vi "TestExec.Route Check Dialog.vi"(8 "Enable Maint":bool, 10 "This Station's Name":string, 11 "Sta Config File":path) -> ()   [LabVIEW 2018]
uses:
  <vilib>/KATE/Files/File Utils.lvlib
panel:
  out "error IO":errorcluster
  out "Main Tab":enum32{"Operate", "Maint"}(tab)
  out "Active":bool
  out "Status":string
  out "Inbound Process Step":string
  in  "SN":string
  in  "Check Route":bool
  in  "Close":bool
  in  "Go To Maint Tab":bool
  in  "ParamName":string="@SN"
  in  "Go To Route Check tab":bool
  in  "This Station's Route List":string[](array[string])
  in  "Load":bool
  in  "Save As":bool
  in  "Save":bool
  in  "Route Config File":path
  in  "Open Route Config":bool
  in  "Open Station Config":bool
  # "UUT Route Check Utility"
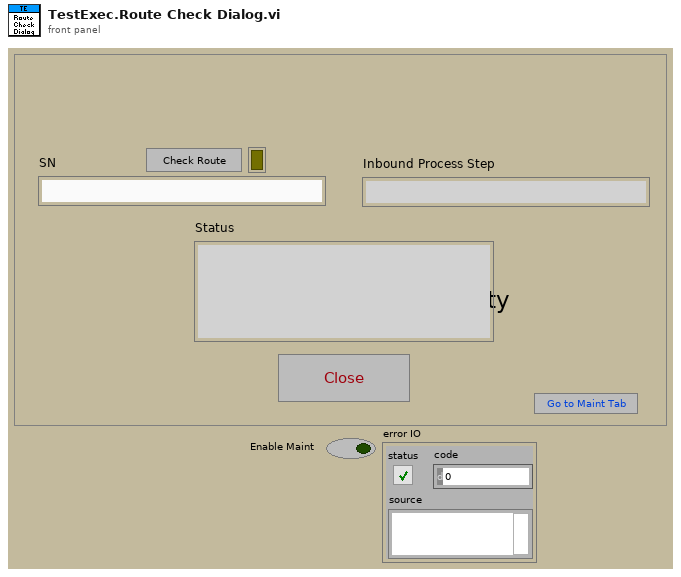
[diagram p1: front panel]
types:
  T1 = enum32{"invalid app kind", "Development System", "Run Time System", "Student Edition", "Embedded LabVIEW", "Evaluation", "Custom"}
  T2 = enum32{"Invalid", "Standard", "Closed", "Hidden", "Minimized", "Maximized"}
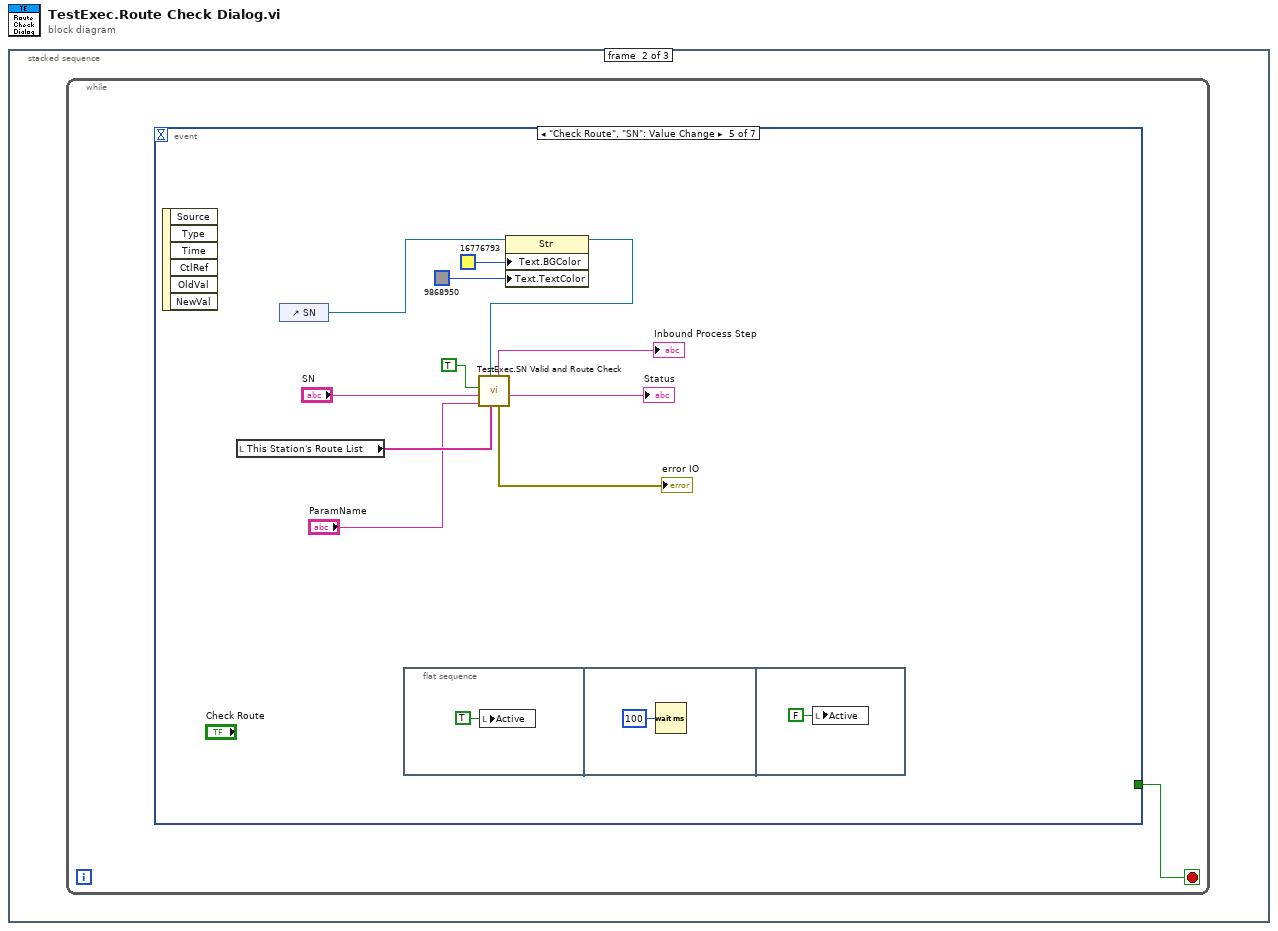
[diagram p0: block diagram]
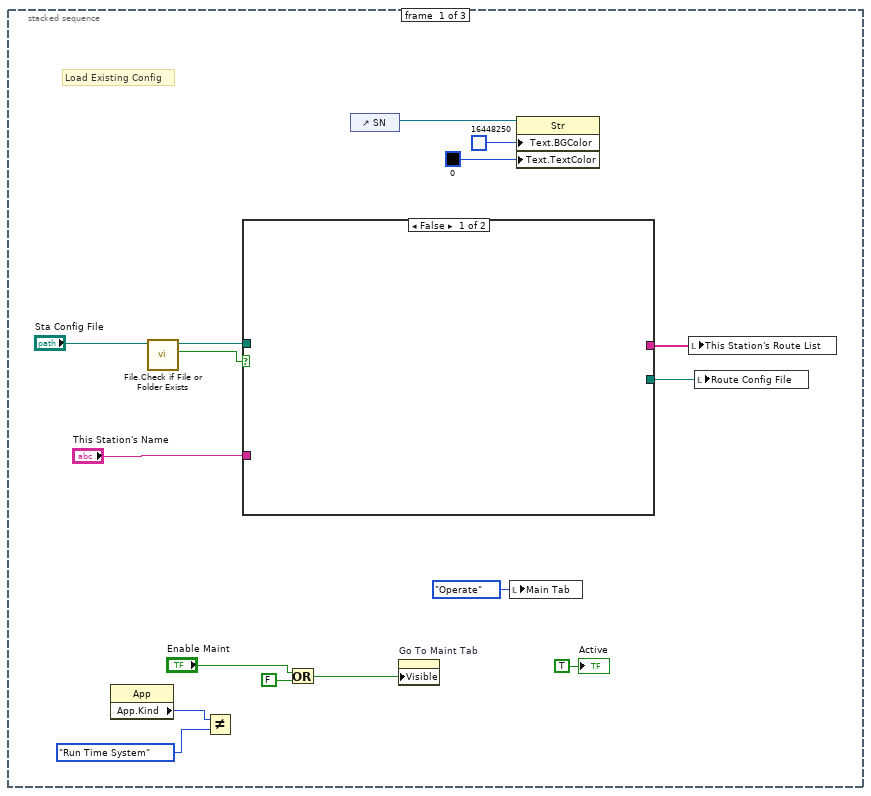
[diagram p2: hidden frame]
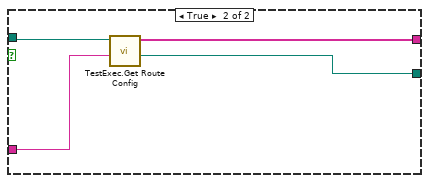
[diagram p3: hidden frame]
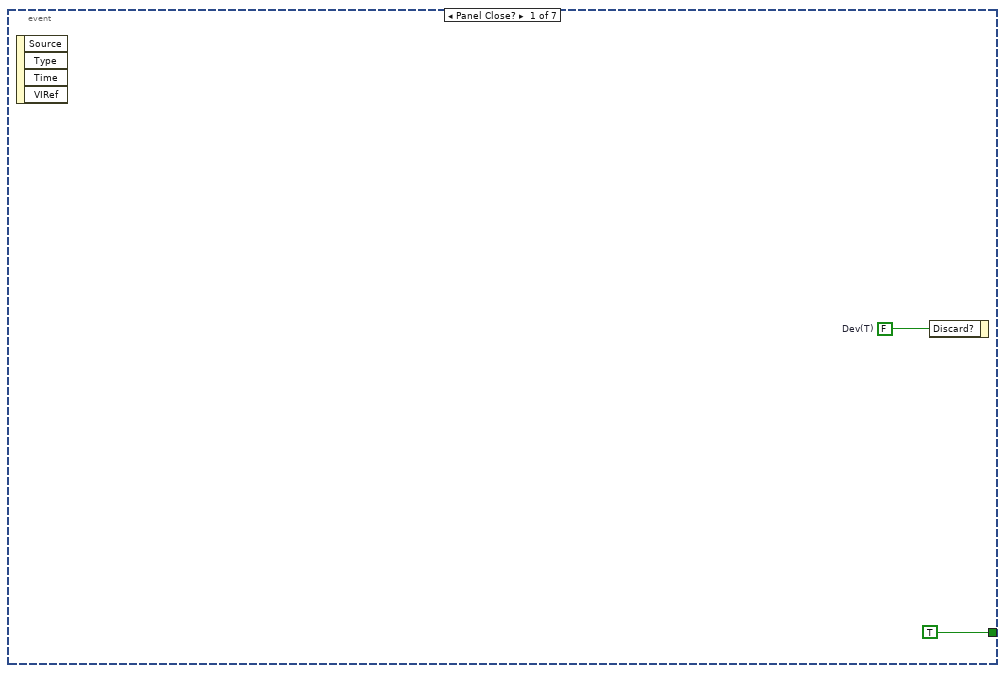
[diagram p4: hidden frame]
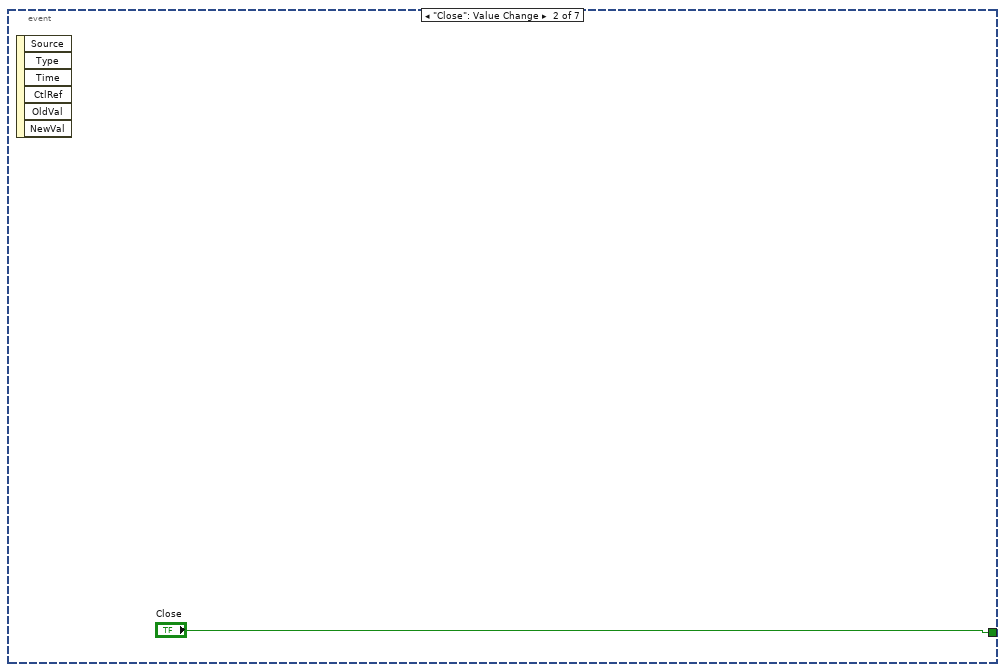
[diagram p5: hidden frame]
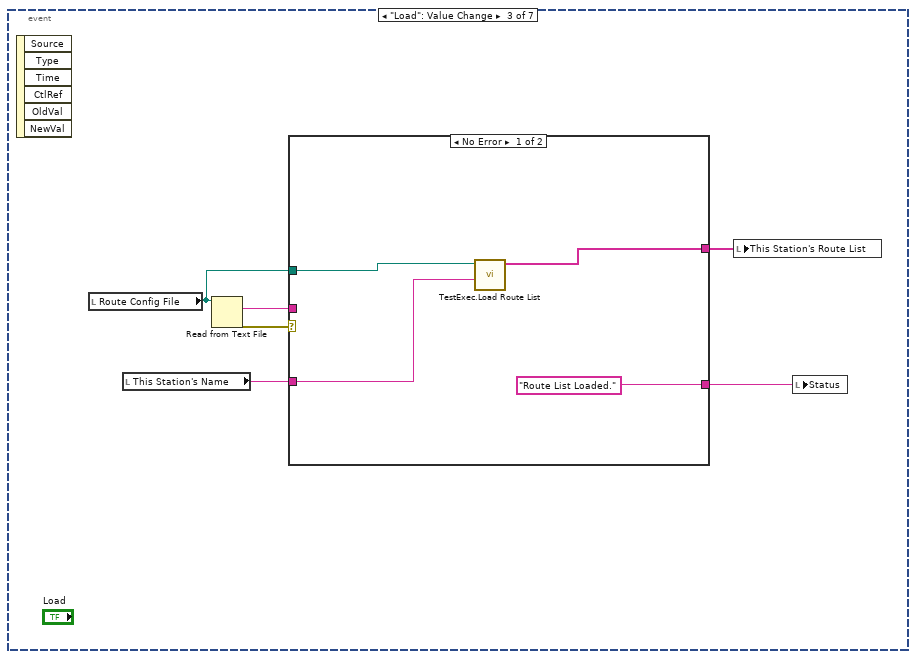
[diagram p6: hidden frame]
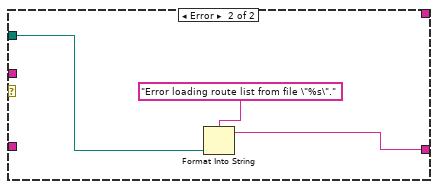
[diagram p7: hidden frame]
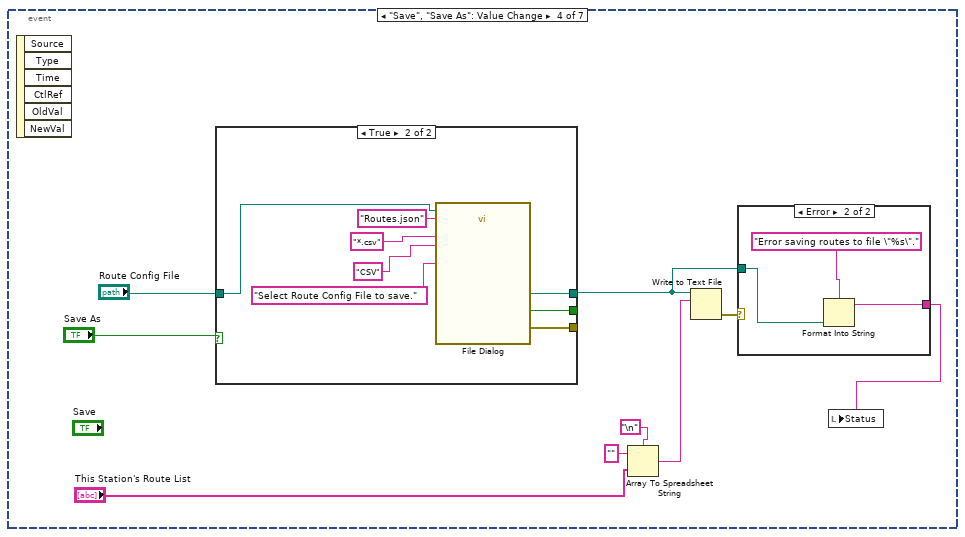
[diagram p8: hidden frame]
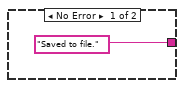
[diagram p9: hidden frame]
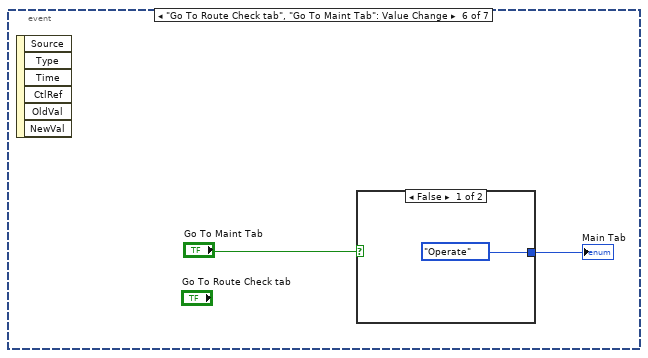
[diagram p11: hidden frame]
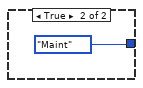
[diagram p12: hidden frame]
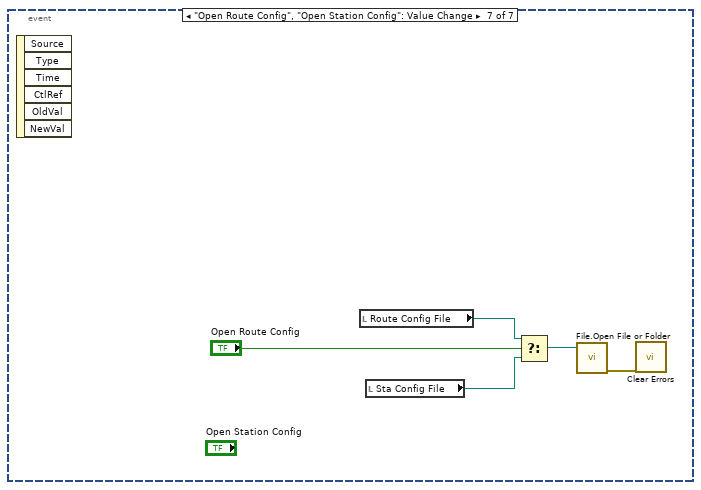
[diagram p13: hidden frame]
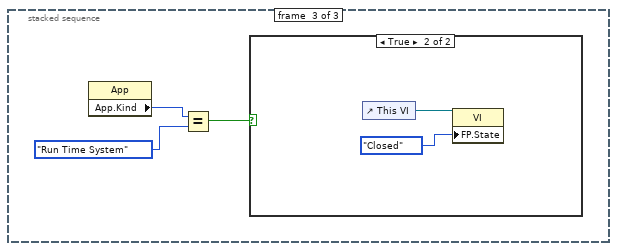
[diagram p14: hidden frame]
diagram:
  n1 = stacked-sequence {
    frame #0 {
      # "Load Existing Config"
      n2 = property class="App"() -> ("App.Kind"=w5:T1)  [unwired: 2 in, 2 out]
      n3 = call <vilib>:"File.Check if File or Folder Exists.vi"("Path"="Sta Config File") -> ("Exists"=w14:bool, "Dup Path"=w15:path)  [unwired: 6 in, 3 out]
      n4 = Not Equal?(x=w5, y=T1."Run Time System" ("Application:Kind")) -> ()  [unwired: 1 out]
      n5 = case shown="False" w14 {
        tunnel: w15 -> [_ w20]
        tunnel: [_ w19] -> w13
        tunnel: [_ w18] -> w12
        tunnel: "This Station's Name" -> [_ w17]
        frame False {
        }
        frame True {
          n6 = call "TestExec.Get Route Config.vi"("Station Name"=w17, "Sta Config INI"=w20) -> ("Route File"=w19:path, "Routes"=w18:string[])  [unwired: 7 in, 1 out]
        }
      }
      n7 = Or(x="Enable Maint", y=FALSE) -> (x .or. y?=w3:bool)
      n8 = control-ref of="SN"() -> (w9:refnum<vi>)
      n9 = property on="Go To Maint Tab" class="Bool"("Visible"=w3) -> ()  [unwired: 2 in, 2 out]
      n10 = local write "Main Tab"(enum32{"Operate", "Maint"}."Operate" ("Main Tab")) -> ()
      n11 = property class="Str"(reference=w9, "Text.BGColor"=u32 16448250, "Text.TextColor"=u32 0) -> ()  [unwired: 1 in, 2 out]
      n12 = local write "This Station's Route List"(w12) -> ()
      n13 = local write "Route Config File"(w13) -> ()
      "Active" <- TRUE ("Active")
    }
    frame #1 {
      n14 = while {
        stop <- w21 stop-if-true
        n15 = event shown="[4] \"Check Route\", \"SN\": Value Change" {
          selector: _ -> [_ _ _ _ _ _ _]
          dyn-events: _ -> [_ _ _ _ _ _ _]
          timeout: _ -> [_ _ _ _ _ _ _]
          tunnel: [TRUE "Close" _ _ _ _ _] -> w21
          event Panel Close? {
            w22 = FALSE  # Dev(T)
            n16 = event-data() -> ()  [unwired: 1 in, 4 out]
            n17 = event-data("Discard?"=w22) -> ()  [unwired: 1 in, 1 out]
          }
          event "Close": Value Change {
            n18 = event-data() -> ()  [unwired: 1 in, 6 out]
          }
          event "Load": Value Change {
            n19 = event-data() -> ()  [unwired: 1 in, 6 out]
            n20 = local read "Route Config File"() -> (w26:path)
            n21 = local read "This Station's Name"() -> (w25:string)
            n22 = Read from Text File(file (use dialog)=w26) -> (text=w30:string, error out=w28:errorcluster)  [unwired: 3 in, 2 out]
            n23 = case shown="No Error" w28 {
              tunnel: w30 -> [_ _]
              tunnel: [w33 _] -> w29
              tunnel: ["Route List Loaded." w36] -> w27
              tunnel: w26 -> [w32 w35]
              tunnel: w25 -> [w31 _]
              frame No Error {
                n24 = call "TestExec.Load Route List.vi"("Station Name"=w31, "Route List File"=w32) -> ("Route List"=w33:string[])  [unwired: 9 in]
              }
              frame Error {
                n25 = Format Into String(format string="Error loading route list from file \"%s\".", w35) -> (resulting string=w36:string)  [unwired: 2 in, 1 out]
              }
            }
            n26 = local write "This Station's Route List"(w29) -> ()
            n27 = local write "Status"(w27) -> ()
          }
          event "Save", "Save As": Value Change {
            n28 = event-data() -> ()  [unwired: 1 in, 6 out]
            n29 = case shown="True" "Save As" {
              tunnel: [w51 w55] -> w38
              tunnel: "Route Config File" -> [w51 w54]
              tunnel: [_ w53] -> _
              tunnel: [_ w52] -> _
              frame False {
              }
              frame True {
                n30 = call "File Dialog"("start path"=w54, "prompt"="Select Route Config File to save." ("prompt (Choose or enter file path)"), "default name"="Routes.json", "pattern (all files)"="*.csv", "pattern label"="CSV" ("pattern (all files)")) -> ("selected path"=w55:path, "cancelled"=w53:bool, "error out"=w52:errorcluster)  [unwired: 7 in, 1 out]
              }
            }
            n31 = Array To Spreadsheet String(delimiter (Tab)="\n", array="This Station's Route List", 3:"" ("format string")) -> (spreadsheet string=w41:string)
            n32 = Write to Text File(file (use dialog)=w38, text=w41) -> (error out=w40:errorcluster)  [unwired: 2 in, 2 out]
            n33 = case shown="Error" w40 {
              tunnel: ["Saved to file." w48] -> w39
              tunnel: w38 -> [_ w49]
              frame No Error {
              }
              frame Error {
                n34 = Format Into String(format string="Error saving routes to file \"%s\".", w49) -> (resulting string=w48:string)  [unwired: 2 in, 1 out]
              }
            }
            n35 = local write "Status"(w39) -> ()
          }
          event "Check Route", "SN": Value Change {
            n36 = event-data() -> ()  [unwired: 1 in, 6 out]
            n37 = local read "This Station's Route List"() -> (w70:string[])
            n38 = control-ref of="SN"() -> (w62:refnum<vi>)
            n39 = flat-sequence {
              frame #0 {
                n40 = local write "Active"(TRUE ("Active")) -> ()
              }
              frame #1 {
                n41 = Wait (ms)(milliseconds to wait=u32 100) -> ()  [unwired: 1 out]
              }
              frame #2 {
                n42 = local write "Active"(FALSE ("Active")) -> ()
              }
            }
            n43 = property class="Str"(reference=w62, "Text.BGColor"=u32 16776793, "Text.TextColor"=u32 9868950) -> (reference out=w61:refnum<vi>)  [unwired: 1 in, 1 out]
            n44 = call "TestExec.SN Valid and Route Check.vi"("Process Steps"=w70, "SN Indicator"=w61, "ParamName"="ParamName", "SN"="SN", "Route Check"=TRUE) -> ("Message"=→"Status":string, "error IO"=→"error IO":errorcluster, "Inbound Process Step"=→"Inbound Process Step":string)  [unwired: 3 in, 1 out]
          }
          event "Go To Route Check tab", "Go To Maint Tab": Value Change {
            n45 = event-data() -> ()  [unwired: 1 in, 6 out]
            n46 = case shown="False" "Go To Maint Tab" {
              tunnel: [enum32{"Operate", "Maint"}."Operate" ("Main Tab") enum32{"Operate", "Maint"}."Maint" ("Main Tab")] -> w75
              frame False {
              }
              frame True {
              }
            }
            "Main Tab" <- w75
          }
          event "Open Route Config", "Open Station Config": Value Change {
            n47 = event-data() -> ()  [unwired: 1 in, 6 out]
            n48 = local read "Route Config File"() -> (w81:path)
            n49 = local read "Sta Config File"() -> (w82:path)
            n50 = Select(t=w81, s="Open Route Config", f=w82) -> (s? t:f=w79:path)
            n51 = call <vilib>:"File.Open File or Folder.vi"("Path"=w79) -> ("Error Out"=w78:errorcluster)  [unwired: 10 in]
            n52 = call <vilib>:"Clear Errors.vi"("error in (no error)"=w78) -> ()  [unwired: 5 in, 2 out]
          }
        }
      }
    }
    frame #2 {
      n53 = property class="App"() -> ("App.Kind"=w83:T1)  [unwired: 2 in, 2 out]
      n54 = property class="App"() -> ("App.Kind"=w87:T1)  [unwired: 2 in, 2 out]
      n55 = Equal?(x=w83, y=T1."Run Time System" ("Application:Kind")) -> ()  [unwired: 1 out]
      n56 = Equal?(x=w87, y=T1."Run Time System" ("Application:Kind")) -> (x = y?=w85:bool)
      n57 = case shown="True" w85 {
        frame False {
        }
        frame True {
          n58 = control-ref of="This VI"() -> (w89:refnum<vi>)
          n59 = property class="VI"(reference=w89, "FP.State"=T2."Closed" ("Front Panel Window:State")) -> ()  [unwired: 1 in, 2 out]
        }
      }
    }
  }
